vi "ROS_parse_LaserScan.vi"(11 "msg in":string) -> (1 "msg_out":string, 2 "LaserScan_msg":T1)   [LabVIEW 2017]
doc: "Parse ROS message type /LaserScan into a cluster"
uses:
  LaserScan.ctl
  <vilib>/Tufts CEEO ROS for LabVIEW Software/ROS/MessageParsing/std_msgs/subs/parse_float32_scalar.vi
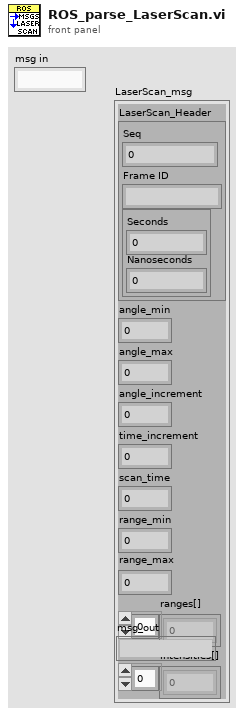
[diagram p1: front panel]
types:
  T1 = typedef "LaserScan.ctl" = cluster{"LaserScan_Header":cluster{"Seq":u32, "Frame ID":string, cluster{"Seconds":i32, "Nanoseconds":i32}}, "angle_min":dbl, "angle_max":dbl, "angle_increment":dbl, "time_increment":dbl, "scan_time":dbl, "range_min":dbl, "range_max":dbl, "ranges[]":dbl[], "intensities[]":dbl[]}
  T2 = cluster{"Seq":u32, "Frame ID":string, "Timestamp":cluster{"Seconds":i32, "Nanoseconds":i32}}
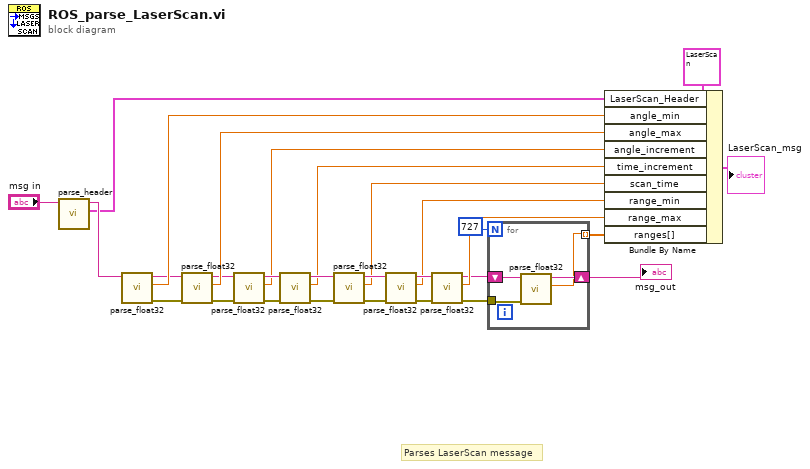
[diagram p0: block diagram]
diagram:
  # "Parses LaserScan message"
  n1 = call <vilib>:"parse_header.vi"("msg in"="msg in") -> ("Header"=w1:T2, "msg out"=w15:string)  [unwired: 4 in, 1 out]
  n2 = call-poly <vilib>:"parse_float32.vi"("msg in"=w15) -> ("error out"=w10:errorcluster, "number"=w17:sgl, "msg out"=w9:string)  [unwired: 4 in]
  n3 = call-poly <vilib>:"parse_float32.vi"("error in"=w10, "msg in"=w9) -> ("error out"=w11:errorcluster, "number"=w18:sgl, "msg out"=w12:string)  [unwired: 3 in]
  n4 = call-poly <vilib>:"parse_float32.vi"("error in"=w11, "msg in"=w12) -> ("error out"=w13:errorcluster, "number"=w19:sgl, "msg out"=w25:string)  [unwired: 3 in]
  n5 = call-poly <vilib>:"parse_float32.vi"("error in"=w13, "msg in"=w25) -> ("error out"=w20:errorcluster, "number"=w21:sgl, "msg out"=w26:string)  [unwired: 3 in]
  n6 = call-poly <vilib>:"parse_float32.vi"("error in"=w20, "msg in"=w26) -> ("error out"=w22:errorcluster, "number"=w23:sgl, "msg out"=w27:string)  [unwired: 3 in]
  n7 = call-poly <vilib>:"parse_float32.vi"("error in"=w22, "msg in"=w27) -> ("error out"=w24:errorcluster, "number"=w6:sgl, "msg out"=w28:string)  [unwired: 3 in]
  n8 = call-poly <vilib>:"parse_float32.vi"("error in"=w24, "msg in"=w28) -> ("error out"=w8:errorcluster, "number"=w7:sgl, "msg out"=w3:string)  [unwired: 3 in]
  n9 = for {
    N: 727 -> [_]
    tunnel: w8 -> [w33]
    shift-right: [w32] -> w4
    shift-left: w3 -> [w31]
    tunnel: [w30] -> w2 mode=indexing
    n10 = call-poly <vilib>:"parse_float32.vi"("error in"=w33, "msg in"=w31) -> ("number"=w30:sgl, "msg out"=w32:string)  [unwired: 3 in, 1 out]
  }
  "msg_out" <- w4
  n11 = Bundle By Name(cluster=T1 {"LaserScan_Header"={"Seq"=0, "Frame ID"="", {"Seconds"=0, "Nanoseconds"=0}}, "angle_min"=0.0, "angle_max"=0.0, "angle_increment"=0.0, "time_increment"=0.0, "scan_time"=0.0, "range_min"=0.0, "range_max"=0.0, "ranges[]"=[], "intensities[]"=[]} ("Cluster"), "LaserScan_Header"=w1, "angle_min"=w17, "angle_max"=w18, "angle_increment"=w19, "time_increment"=w21, "scan_time"=w23, "range_min"=w6, "range_max"=w7, "ranges[]"=w2) -> (→"LaserScan_msg":T1)
